vi "Write Pulse Data Points.vi"(8 "error in":errorcluster, 10 "Data Pts":i32, 11 "3300 in":refnum<class "3300.lvclass">) -> (0 "error out":errorcluster, 3 "3300 out":refnum<class "3300.lvclass">)   [LabVIEW 2019, in "3300.lvlib" / "3300.lvclass"]
uses:
  Library/3300.lvclass
  C:/Users/Public/Documents/Development/builds/Engine/Monitored Actor.lvlibp/Monitored Actor/Monitored Actor/Monitored Actor.lvclass
  builds/Engine/Monitored Actor.lvlibp/Monitored Actor/Monitored Actor/Read Actor Label.vi
  builds/Instruments/Electronic Load.lvlibp/Library/Electronic Load.lvclass
  builds/Engine/Engine.lvlibp/Project/Engine.lvclass
  builds/Instruments/Instruments.lvlibp/Library/Instruments.lvclass
  C:/Users/Public/Documents/Development/builds/Engine/Engine.lvlibp/Project/Engine.lvclass
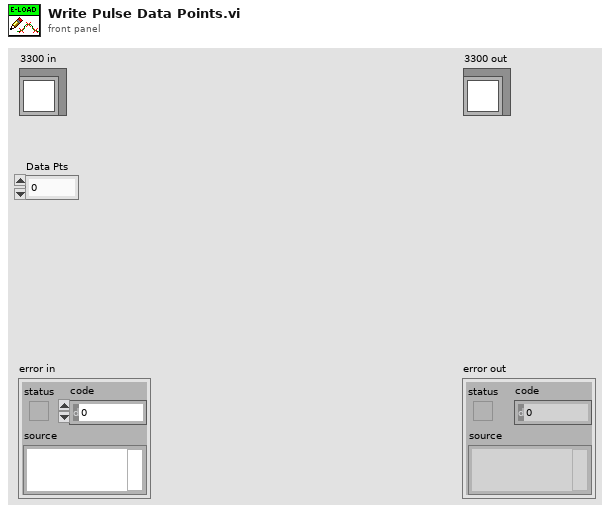
[diagram p1: front panel]
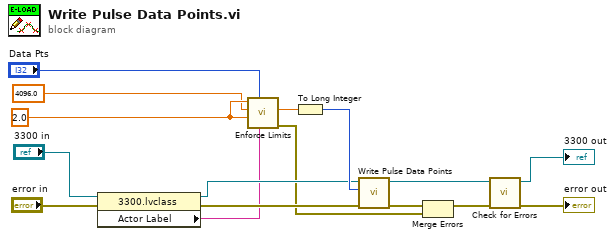
[diagram p0: block diagram]
diagram:
  w2 = 2.0 ("Minimum")
  n1 = property class="3300.lvclass"(reference="3300 in", error in="error in") -> (reference out=w5:refnum<class "3300.lvclass">, error out=w6:errorcluster, "Actor Label"=w4:string)
  n2 = call "Enforce Limits.vi"("Device"=w4, "Setpoint"="Data Pts", "Minimum"=w2, "Maximum"=4096.0 ("Previous"), "Previous"=w2) -> ("error out"=w3:errorcluster, "Protected Setpoint"=w12:dbl)  [unwired: 5 in]
  n3 = To Long Integer(number=w12) -> (32bit integer=w11:i32)
  n4 = call-parent "Write Pulse Data Points.vi"("error in"=w6, "Data Pts"=w11, "Electronic Load in"=w5) -> ("error out"=w10:errorcluster, "Electronic Load out"=w16:refnum<class "3300.lvclass">)  [unwired: 7 in]
  n5 = Merge Errors(w10, w3) -> (w9:errorcluster)
  n6 = call "Check for Errors.vi"("error in"=w9, "Engine in"=w16) -> ("error out"=→"error out":errorcluster, "Engine out"=→"3300 out":refnum<class "3300.lvclass">)  [unwired: 8 in]
